vi "MT Apply Fading Profile.vi"   [LabVIEW 2020, in "niDMT.lvlib"]
doc: "Applies a fading profile to fade the complex baseband modulated waveform. The faded waveform can be used to test receiver immunity to fading channels."
uses:
  <vilib>/addons/Modulation/niDMT.lvlib
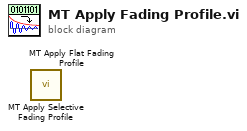
[diagram p0: block diagram]
diagram:
  n1 = call <vilib>:"MT Apply Selective Fading Profile.vi"() -> ()  [unwired: 14 in, 2 out]
  n2 = call <vilib>:"MT Apply Flat Fading Profile.vi"() -> ()  [unwired: 14 in, 2 out]
